vi "Configure Glitch Trigger Range.vi"(8 "error in (no error)":errorcluster {"code" format="%.0x"}, 9 "lower (20.0E-9 sec)":dbl=2e-08 caption="Lower (20.0E-9 sec)" format="%^.2e", 10 "upper (30.0E-9 sec)":dbl=3e-08 caption="Upper (30.0E-9 sec)" format="%^.2e", 11 "VISA Resource Name":refnum<visa-resource-name>) -> (0 "error out":errorcluster {"code" format="%.0x"}, 3 "VISA Resource Name Out":refnum<visa-resource-name>)   [LabVIEW 2011, in "Agilent 546XX Series.lvlib"]
doc: "This VI specifies the glitch width range values. A glitch trigger occurs when the trigger signal has a pulse with a width that is less than the upper glitch width range value and greater than the lower glitch width range value. \n\nNotes: \n\n(1) This VI affects instrument behavior only if the trigger type is set to Glitch Trigger and the Glitch Condition is set to Within Range. Call the ag546xx Configure Trigger and ag546xx Configure Glitch Trigger Source VIs to set the trigger type and glitch trigger condition before calling this VI."
uses:
  Agilent 546XX Series.lvlib
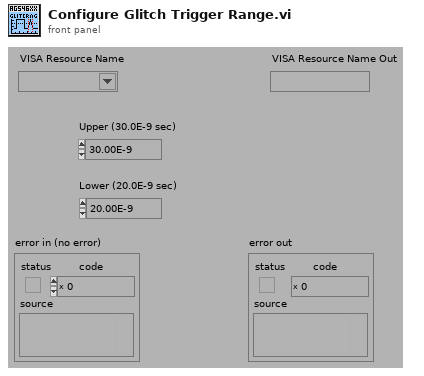
[diagram p1: front panel]
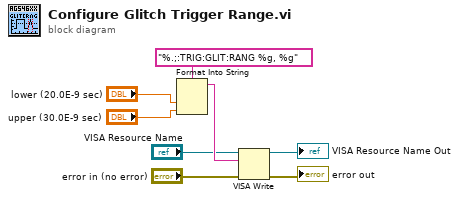
[diagram p0: block diagram]
diagram:
  n1 = Format Into String(format string="%.;:TRIG:GLIT:RANG %g, %g", "lower (20.0E-9 sec)", "upper (30.0E-9 sec)") -> (resulting string=w5:string)  [unwired: 2 in, 1 out]
  n2 = VISA Write(VISA resource name="VISA Resource Name", write buffer=w5, error in (no error)="error in (no error)") -> (VISA resource name out=→"VISA Resource Name Out":refnum<visa-resource-name>, error out=→"error out":errorcluster)  [unwired: 1 out]
